vi "Solution Handle Errors.vi"() -> ()   [LabVIEW 2019]
uses:
  <vilib>/Utility/error.llb/DialogType.ctl
panel:
  out "Text from File":string
  in  "File Path":path=path "C:/Users/Barron Stone/Desktop/Exercise Files/CH06/06_06/end/digits.txt"
  # "NOTE: Use the browse button to select the file path\nto \"digits.txt\" on your own computer."
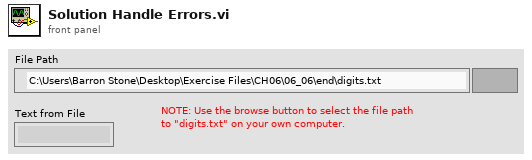
[diagram p1: front panel]
types:
  T1 = typedef "DialogType.ctl" = u16
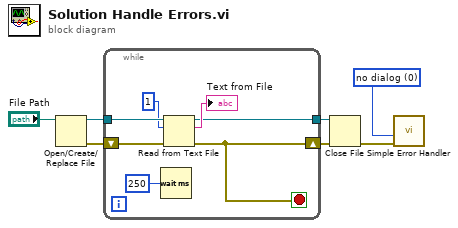
[diagram p0: block diagram]
diagram:
  w1 = T1 0 items=["no dialog", "OK message", "continue or stop message", "OK message + warnings", "continue/stop + warnings"] ("type of dialog (OK msg:1)")
  n1 = Open/Create/Replace File(file path (use dialog)="File Path") -> (refnum out=w6:refnum<file>, error out=w4:errorcluster)  [unwired: 5 in, 1 out]
  n2 = while {
    tunnel: w6 -> [w14]
    tunnel: [w12] -> w5
    shift-right: [w8] -> w3
    shift-left: w4 -> [w9]
    stop <- w8 stop-if-true
    n3 = Wait (ms)(milliseconds to wait=u32 250) -> ()  [unwired: 1 out]
    n4 = Read from Text File(file (use dialog)=w14, count=1, error in=w9) -> (refnum out=w12:refnum<file>, text=→"Text from File":string, error out=w8:errorcluster)  [unwired: 1 in, 1 out]
  }
  n5 = Close File(refnum=w5, error in=w3) -> (error out=w2:errorcluster)  [unwired: 1 out]
  n6 = call <vilib>:"Simple Error Handler.vi"("type of dialog (OK msg:1)"=w1, "error in (no error)"=w2) -> ()  [unwired: 3 in, 5 out]
